vi "Time_Auto.vi"(9 "Sample_Time":u32, 10 "Counter":i32, 11 "Time_to_wait":i32) -> (3 "Boolean":bool)   [LabVIEW 2015]
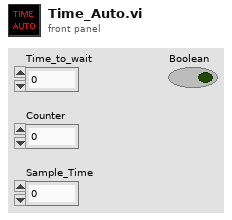
[diagram p1: front panel]
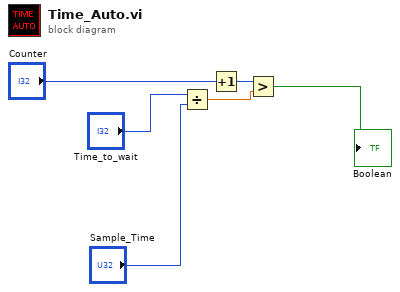
[diagram p0: block diagram]
diagram:
  n1 = Divide(x="Time_to_wait", y="Sample_Time") -> (x/y=w4:dbl)
  n2 = Increment(x="Counter") -> (x+1=w3:i32)
  n3 = Greater?(x=w3, y=w4) -> (0:→"Boolean":bool)
